vi "Text File Data Extraction.vi"(11 "File Path Input":path) -> (0 "error out":errorcluster, 2 "Array":dbl[][](array[numeric]), 3 "File Path Output":path)   [LabVIEW 2014]
panel:
  # "Text File Data Extraction"
  # "Inputs"
  # "Outputs"
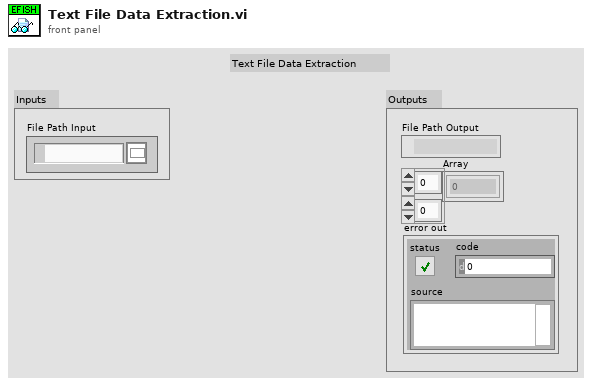
[diagram p1: front panel]
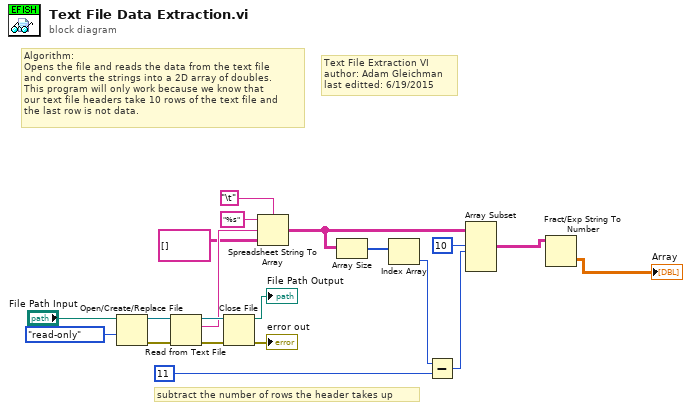
[diagram p0: block diagram]
diagram:
  # "Algorithm:\nOpens the file and reads the data from the text file\nand converts the strings into a 2D array of doubles.\nThis program will only work because we know that \nour text file headers take 10 rows of the text file and\nthe last row is not data."
  # "Text File Extraction VI\nauthor: Adam Gleichman\nlast editted: 6/19/2015"
  # "subtract the number of rows the header takes up"
  n1 = Open/Create/Replace File(file path (use dialog)="File Path Input", access (0:read/write)=enum16{"read/write", "read-only", "write-only"}."read-only") -> (refnum out=w18:refnum<file>, error out=w17:errorcluster)  [unwired: 4 in, 1 out]
  n2 = Read from Text File(file (use dialog)=w18, error in=w17) -> (refnum out=w16:refnum<file>, text=w13:string, error out=w15:errorcluster)  [unwired: 2 in, 1 out]
  n3 = Close File(refnum=w16, error in=w15) -> (path=→"File Path Output":path, error out=→"error out":errorcluster)
  n4 = Spreadsheet String To Array(delimiter (Tab)="\t", format string="%s", spreadsheet string=w13, array type (2D Dbl)=string[][] []) -> (array=w6:string[][])
  n5 = Array Size(array=w6) -> (size(s)=w9:i32[])
  n6 = Index Array(array=w9) -> (element=w8:i32)  [unwired: 1 in]
  n7 = Subtract(x=w8, y=11) -> (x-y=w4:i32)
  n8 = Array Subset(array=w6, index (row)=10 ("index"), length (row)=w4) -> (w2:string[][])  [unwired: 2 in]
  n9 = Fract/Exp String To Number(string=w2) -> (number=→"Array":dbl[][])  [unwired: 3 in, 1 out]
